vi "Number of LBCBs 2 Window Size.vi"(0 "Number of\nLBCBs Out":T1, 1 "Rigid Connection In":bool) -> (2 "Combined Visible":bool, 3 "Window Size":i32, 4 "LBCB 2 Visible":bool)   [LabVIEW 2013]
uses:
  Data Access Objects/Application/Number Of LBCBs.ctl
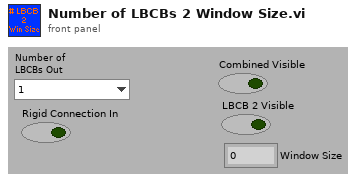
[diagram p1: front panel]
types:
  T1 = typedef "Number Of LBCBs.ctl" = enum16{"1", "2"}
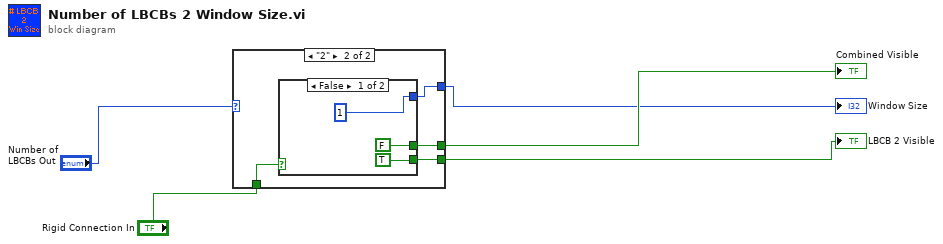
[diagram p0: block diagram]
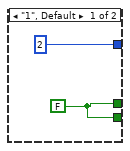
[diagram p2: hidden frame]
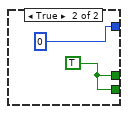
[diagram p3: hidden frame]
diagram:
  n1 = case shown="\"2\"" "Number of\nLBCBs Out" {
    tunnel: "Rigid Connection In" -> [_ w11]
    tunnel: [2 w10] -> w3
    tunnel: [w6 w9] -> w4
    tunnel: [w6 w8] -> w5
    frame "1", Default {
      w6 = FALSE
    }
    frame "2" {
      n2 = case shown="False" w11 {
        tunnel: [1 ("f") 0] -> w10
        tunnel: [FALSE w15] -> w9
        tunnel: [TRUE w15] -> w8
        frame False {
        }
        frame True {
          w15 = TRUE
        }
      }
    }
  }
  "LBCB 2 Visible" <- w5
  "Combined Visible" <- w4
  "Window Size" <- w3
